vi "JoystickRumble.vi"(0 "Rumble":bool) -> ()   [LabVIEW 2018]
uses:
  <vilib>/Rock Robotics/WPI/Utilities/WPI_GetSetVariantRefNum.vi
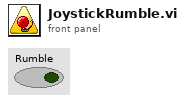
[diagram p1: front panel]
types:
  T1 = typedef "WPI_JoystickDevRef.ctl" = cluster{"Device":T2}
  T2 = typedef "WPI_JoystickDeviceEnum.ctl" = enum16{"USB 0", "USB 1", "USB 2", "USB 3", "USB 4", "USB 5"}
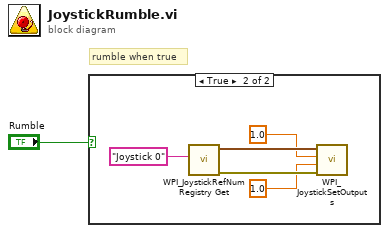
[diagram p0: block diagram]
diagram:
  # "rumble when true"
  n1 = case shown="True" "Rumble" {
    frame False {
    }
    frame True {
      n2 = call <vilib>:"WPI_JoystickRefNum Registry Get.vi"("refnum name"="Joystick 0") -> ("error out"=w5:errorcluster, "JoystickDevRef"=w6:T1)  [unwired: 1 in, 8 out]
      n3 = call <vilib>:"WPI_JoystickSetOutputs.vi"("error in (no error)"=w5, "Right Rumble"=sgl 1.0, "Left Rumble"=sgl 1.0, "JoystickDevRef"=w6) -> ()  [unwired: 6 in, 2 out]
    }
  }
